vi "Main Swerve Loop.vi"() -> ()   [LabVIEW 2020]
doc: "Controls the Swerve Drive Subsytem.\nAll loops containing the calculation and implementation of Swerve Drive are self-contained within this vi.\nPlace this vi in Periodic Tasks."
uses:
  <vilib>/Rock Robotics/WPI/ThirdParty/Sensors/navX/_TypeDefs/FRIC_navX_DeviceNumbersTypeDef.ctl
  Swerve Global Variables.vi
panel:
  in  "PID gains":T1={"proportional gain (Kc)"=0.04, "integral time (Ti, min)"=0.0, "derivative time (Td, min)"=0.0} {"proportional gain (Kc)" format="%_6f"; "integral time (Ti, min)" format="%_6f"; "derivative time (Td, min)" format="%_6f"}
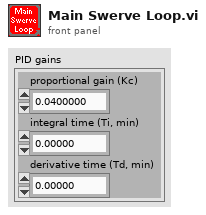
[diagram p1: front panel]
types:
  T1 = cluster{"proportional gain (Kc)":dbl, "integral time (Ti, min)":dbl, "derivative time (Td, min)":dbl}
  T2 = typedef "FRIC_navX_DeviceNumbersTypeDef.ctl" = enum16{"Dev0", "Dev1", "Dev2", "Dev3"}
  T3 = cluster{"Yaw":dbl, "Roll":dbl, "Pitch":dbl, "Heading":dbl, "Fused Heading":dbl}
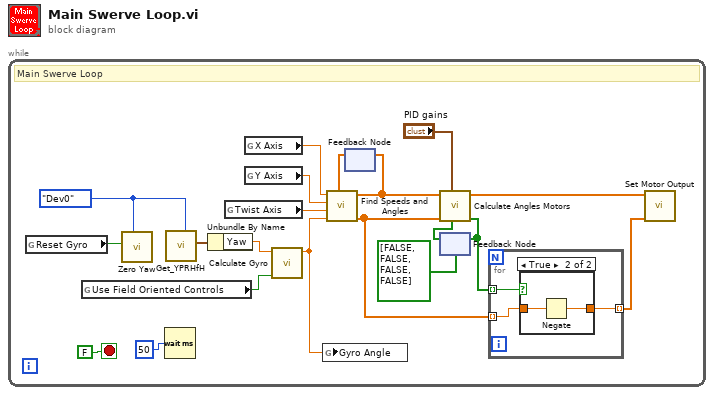
[diagram p0: block diagram]
diagram:
  n1 = while {
    stop <- FALSE stop-if-true
    w7 = FRIC_navX_DeviceNumbersTypeDef."Dev0" ("Device Number")
    # "Main Swerve Loop"
    n2 = global read "Swerve Global Variables.vi" "Reset Gyro"() -> (w8:bool)
    n3 = global read "Swerve Global Variables.vi" "Use Field Oriented Controls"() -> (w19:bool)
    n4 = call <vilib>:"Zero Yaw.vi"("Device Number"=w7, "Zero"=w8) -> ()  [unwired: 10 in]
    n5 = Wait (ms)(milliseconds to wait=u32 50) -> ()  [unwired: 1 out]
    n6 = call <vilib>:"Get_YPRHfH.vi"("Device Number"=w7) -> ("YRPHfH"=w10:T3)  [unwired: 10 in]
    n7 = Unbundle By Name(w10) -> ("Yaw"=w9:dbl)
    n8 = global read "Swerve Global Variables.vi" "Twist Axis"() -> (w17:dbl)
    n9 = global read "Swerve Global Variables.vi" "X Axis"() -> (w20:dbl)
    n10 = global read "Swerve Global Variables.vi" "Y Axis"() -> (w18:dbl)
    n11 = call "Calculate Gyro.vi"("Field Oriented Control?"=w19, "Yaw"=w9) -> ("Gyro Angle"=w1:dbl)  [unwired: 9 in]
    n12 = global write "Swerve Global Variables.vi" "Gyro Angle"(w1) -> ()
    n13 = feedback #1() -> (w13:dbl[])  [unwired: 1 in]
    n14 = call "Find Speeds and Angles.vi"("Prev Angles"=w13, "Gyro Angle"=w1, "Twist Axis"=w17, "Y Axis"=w18, "X Axis"=w20) -> ("Speeds"=w2:dbl[], "Angles"=w4:dbl[])  [unwired: 3 in]
    n15 = feedback-in #1(w4) -> ()
    n16 = feedback #2(bool[] [FALSE, FALSE, FALSE, FALSE] ("Flip Speeds?")) -> (w3:bool[])
    n17 = call "Calculate Angles Motors.vi"("Prev Flip Speeds?"=w3, "PID gains"="PID gains", "Speeds"=w2, "Angles"=w4) -> ("Flip Speeds?"=w14:bool[], "Angle Motor Outputs"=w5:dbl[])  [unwired: 6 in]
    n18 = feedback-in #2(w14) -> ()
    n19 = for {
      tunnel: w14 -> [w23] mode=indexing
      tunnel: [w22] -> w6 mode=indexing
      tunnel: w2 -> [w21] mode=indexing
      n20 = case shown="True" w23 {
        tunnel: [w24 w26] -> w22
        tunnel: w21 -> [w24 w25]
        frame False {
        }
        frame True {
          n21 = Negate(x=w25) -> (-x=w26:dbl)
        }
      }
    }
    n22 = call "Set Motor Output.vi"("Speed Motor Outputs"=w6, "Angle Motor Outputs"=w5) -> ()  [unwired: 10 in]
  }
